vi "lib Create Path If Necessary.vi"(11 "path":path) -> (3 "path out":path)   [LabVIEW 2024]
panel:
  out "error out":errorcluster
  in  "error in (no error)":errorcluster
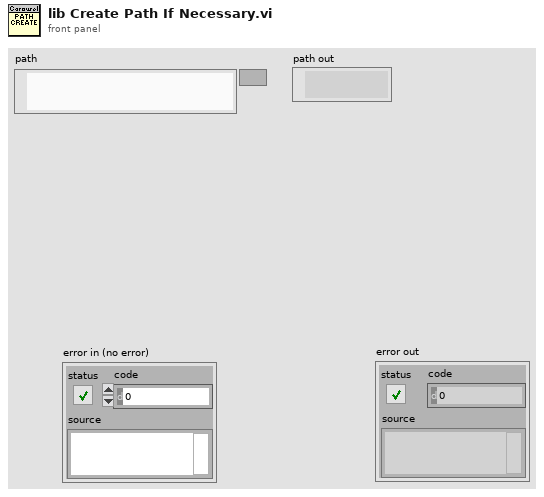
[diagram p1: front panel]
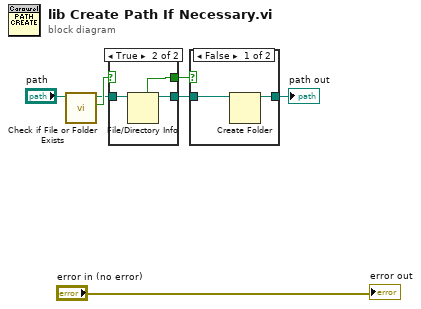
[diagram p0: block diagram]
diagram:
  n1 = call <vilib>:"Check if File or Folder Exists.vi"("path"="path") -> ("file or folder exists?"=w6:bool, "dup path"=w5:path)  [unwired: 8 in, 1 out]
  n2 = case shown="True" w6 {
    selector: w6 -> [w9 _]
    tunnel: w5 -> [w8 w12]
    tunnel: [w9 w11] -> w4
    tunnel: [w8 w10] -> w3
    frame False {
    }
    frame True {
      n3 = File/Directory Info(path=w12) -> (path out=w10:path, directory=w11:bool)  [unwired: 1 in, 5 out]
    }
  }
  n4 = case shown="False" w4 {
    tunnel: w3 -> [w14 w15]
    tunnel: [w13 w15] -> w1
    frame False {
      n5 = Create Folder(path (use dialog)=w14) -> (created path=w13:path)  [unwired: 2 in, 2 out]
    }
    frame True {
    }
  }
  "path out" <- w1
  "error out" <- "error in (no error)"
